vi "number5-sub4.vi"(4 "Array 2":i32[](array[numeric]), 5 "index (page)":i32, 6 "Array 3":bool[][][](array[boolean])) -> (2 "output array":bool[][][](array[boolean]))   [LabVIEW 2014]
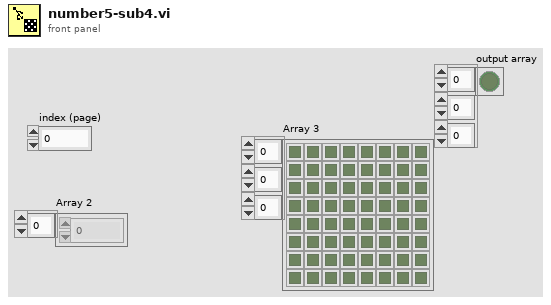
[diagram p1: front panel]
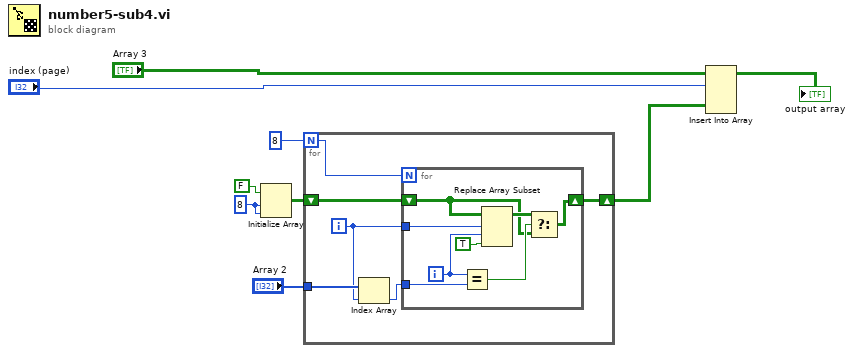
[diagram p0: block diagram]
diagram:
  w8 = 8
  n1 = Initialize Array(FALSE, w8, w8) -> (w7:bool[][])
  n2 = for {
    N: 8 -> [w15]
    shift-right: [w10] -> w2
    shift-left: w7 -> [w14]
    tunnel: "Array 2" -> [w13]
    i -> [w11]
    n3 = Index Array(array=w13, index=w11) -> (element=w12:i32)
    n4 = for {
      N: w15 -> [_]
      shift-right: [w18] -> w10
      shift-left: w14 -> [w17]
      tunnel: w12 -> [w23]
      tunnel: w11 -> [w22]
      i -> [w21]
      n5 = Equal?(x=w21, y=w23) -> (x = y?=w19:bool)
      n6 = Replace Array Subset(array=w17, new element=TRUE, index (row)=w22, index (col)=w21) -> (w20:bool[][])
      n7 = Select(t=w20, s=w19, f=w17) -> (s? t:f=w18:bool[][])
    }
  }
  n8 = Insert Into Array(array="Array 3", index (dim 0)="index (page)", new element=w2) -> (→"output array":bool[][][])  [unwired: 2 in]
